vi "Dashboard Main.vi"() -> ()   [LabVIEW 2018]
uses:
  <vilib>/Utility/miscctls.llb/LVRowAndColumnTypeDef.ctl
  <vilib>/event_ctls.llb/eventvkey.ctl
  <vilib>/Rock Robotics/WPI/Dashboard/WPI_DashboardLogging Global.vi
  <vilib>/Rock Robotics/Network Tables/NT Read Boolean Array.vi
  <vilib>/Rock Robotics/Network Tables/NT Read Boolean.vi
panel:
  in  "TCP":refnum<k5>
  out "Robot IP":string
  out "Image Message":string="Timeout in Camera Communications"
  in  "Dashboard Tab":T1(tab)
  out "Boolean 17":bool
  out "Boolean 16":bool
  out "Boolean 15":bool
  out "Boolean 14":bool
  out "Boolean 13":bool
  out "Boolean 12":bool
  out "Boolean 11":bool
  out "Boolean 10":bool
  out "Boolean 9":bool
  out "Boolean 8":bool
  out "Boolean":bool
  out "Boolean":bool
  out "Boolean 6":bool
  out "Boolean 5":bool
  out "Boolean 4":bool
  out "Boolean 3":bool
  out "Boolean 2":bool
  out "Boolean":bool
  out "Elevator\nPosition":cluster{dbl, dbl}(slide) scale=0.0..22000.0
  out "Hatch Open":bool
  out "Hatch Close":bool
  out "Ball Out":bool
  out "Ball In":bool
  in  "Select Auto":string(combo)="Select Autonomous ..."
  out "NT Connection":bool
  out "Mode":T2(ring)=enum."Auto Disabled"
  out "Right Camera Perf":cluster{"Bandwidth (Mbps)":dbl, "FPS":dbl}
  in  "Rec Mode":enum32{"Stop", "Record", "Playback"}(radio)
  in  "Camera Name Right":string(combo)="No Camera Selection"
  in  "Camera Settings Right":T3={"Frame Rate"=30, "Compression"=30, "Size"=1, "DB Camera Config"=FALSE} {"Frame Rate" scale=1.0..30.0; "Compression" scale=100.0..-1.0; "Size" items=["640x480", "320x240", "160x120"]}
  in  "Camera Name":string(combo)="No Camera Selection"
  in  "Camera Settings":T3={"Frame Rate"=30, "Compression"=30, "Size"=1, "DB Camera Config"=FALSE} {"Frame Rate" scale=1.0..30.0; "Compression" scale=100.0..-1.0; "Size" items=["640x480", "320x240", "160x120"]}
  out "Camera Perf":string
  out "Boolean":bool
  out "Camera Image Right":T4(plugin-control)
  in  "DB/String 9":string
  in  "DB/String 8":string
  in  "DB/String 7":string
  in  "DB/String 6":string
  in  "DB/String 5":string
  in  "DB/String 4":string
  in  "DB/String 3":string
  in  "DB/String 2":string
  in  "DB/String 1":string
  in  "DB/String 0":string
  in  "DB/Slider 0":dbl(slide) scale=0.0..5.0
  in  "DB/Slider 1":dbl(slide) scale=0.0..5.0
  in  "DB/Slider 2":dbl(slide) scale=0.0..5.0
  in  "DB/Slider 3":dbl(slide) scale=0.0..5.0
  out "DB/LED 3":bool
  out "DB/LED 2":bool
  out "DB/LED 1":bool
  out "DB/LED 0":bool
  in  "DB/Button 3":bool
  in  "DB/Button 2":bool
  in  "DB/Button 1":bool
  in  "DB/Button 0":bool caption="New Name"
  in  "Test Slider":dbl(slide) scale=0.0..100.0 scale format="%#_3g"
  in  "On/Off":bool caption="Solenoid"
  in  "Test Name":u16(ring) items=["Select the test to run..."]
  in  "Test Tree":string(tree)
  in  "Motor":cluster{"Value":dbl, "Enable":bool} {"Value" scale=-1.0..1.0 scale format="%#_3g"}
  out "Progress":T5 {"Test Progress" scale=0.0..100.0}
  in  "Rev/Fwd":cluster{"Forward":bool, "Reverse":bool}
  in  "Test Ring":u16(ring) items=["Monochrome", "Color"]
  out "Cmd Status":string
  in  "Execute Command":bool
  in  "Command Params":string[][](table)
  in  "Command Selection":i32(listbox)
  in  "CheckList":i32(listbox)
  out "Tree":string(tree)
  out "Camera Image":T4(plugin-control)
  out "Background":bool
  # "Use this one"
  # "HW"
  # "HW"
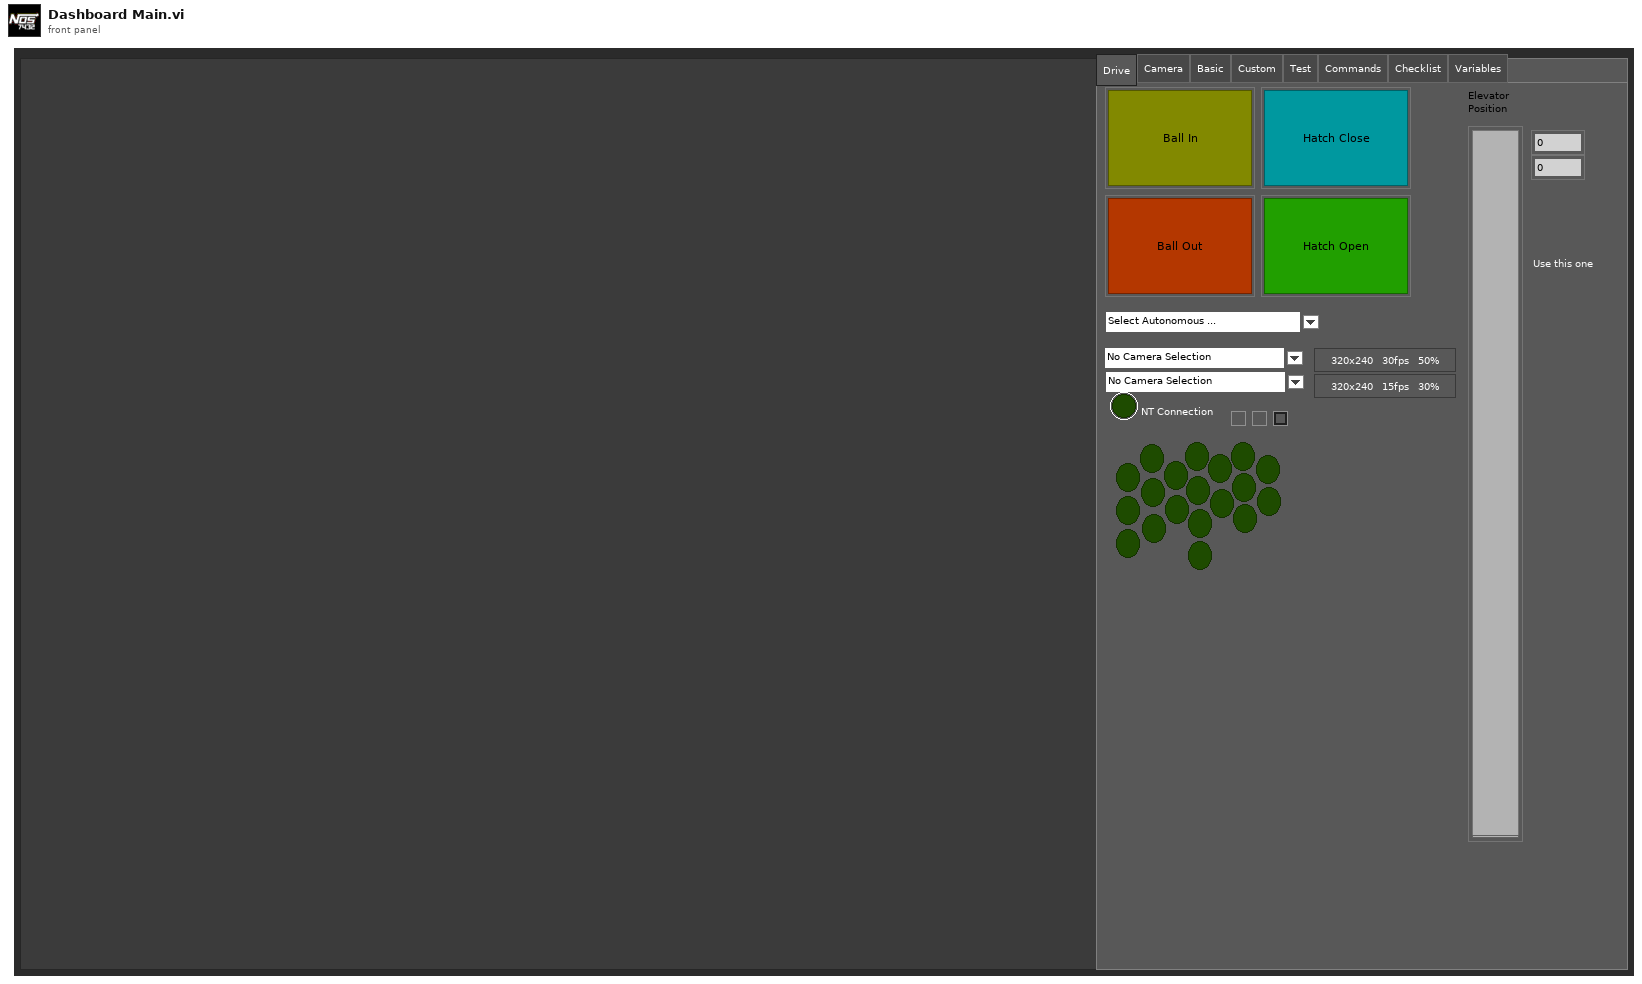
[diagram p1: front panel]
types:
  T1 = enum32{"Drive", "Camera", "Basic", "Custom", "Test", "Commands", "Checklist", "Variables"}
  T2 = enum8{"Tele-Op Disabled", "Tele-Op Enabled", "Auto Disabled", "Auto Enabled", "Test Disabled", "Test Enabled", "Disconnected", "No Code", "E-Stop"}
  T3 = cluster{"Frame Rate":i32, "Compression":i32, "Size":u16, "DB Camera Config":bool}
  T4 = typedef "IMAQ Image.ctl" = refnum<image>
  T5 = cluster{"Test Progress":u8, "Test Progress Text":string}
  T6 = cluster{"Save Path":path, "Interval (s)":dbl, "Keep":i32}
  T7 = typedef "Image Type" = u32
  T8 = cluster{"IDs":cluster{"RPC field ID":u16, "Unique ID":u16}, "String":string}
  T9 = cluster{"Error Strings":string, "Disable Counts":cluster{u16, u16}, "Rail Faults":cluster{u16, u16, u16}, "Robot IP":string, "DB Mode":u8, "Event Info":cluster{"Name":string, "Type":u8, "Number":u16, "Replay":u8}}
  T10 = cluster{"Storage":cluster{"Disk Free":u64, "RAM Block":u32, "RAM free":u32}, "CPU Utilization":cluster{"CPU % ISR":sgl, "CPU % Time Crit":sgl, "CPU % Timed Str":sgl, "CPU % High":sgl, "CPU % Above":sgl, "CPU % Normal":sgl, "CPU % Low":sgl}, "CAN":cluster{"% Bus Utilization":sgl, "Bus Off Cnt":u32, "TX_FIFO Full Cnt":u32, "Receive Error Cnt":u8, "Transmit Error Cnt":u8}, "HID":cluster{"HID Outputs":u32, "Rumble Low":u16, "Rumble High":u16}[]}
  T11 = cluster{"Status bits":cluster{"Test Mode":bool, "Autonomous":bool, "Enabled":bool, "Code Start":bool, "Brownout":bool, "Reserved 2":bool, "Reserved 3":bool, "E-Stop":bool}, "Code Trace":cluster{"Disabled":bool, "TeleOp":bool, "Auto":bool, "Test":bool}, "Controller Type":enum16{"unknown", "cRIO", "roboRio"}, "Code?":enum16{"unknown", "noCode", "code"}, "Battery V":dbl}
  T12 = cluster{"Control Bits":cluster{"TestMode":bool, "Autonomous":bool, "Enabled":bool, "FMS Present":bool, bool, bool, bool, "E-Stop":bool}, "Team Station ":u8, "Countdown":sgl, "Joystick Values":cluster{"Axes":dbl[], "Buttons":bool[], "POVs":i16[]}[]}
  T13 = cluster{"Global Rectangle":i32[], "Contours":cluster{"Contour Type":u32, "ROI Type":u32, "Points":i32[]}[]}
  T14 = cluster{"Camera Name":string, string, "Saved DB Images Info":cluster{"Save Path":path, "Interval (s)":dbl, "Keep":i32}}
  T15 = cluster{"Camera Name Right":string, string, "Saved DB Images Info":cluster{"Save Path":path, "Interval (s)":dbl, "Keep":i32}}
  T16 = cluster{"Operation":enum16{"Update", "Clear"}, "Color Box":u32}[]
  T17 = typedef "eventvkey.ctl" = enum16{"ASCII", "Enter", "Return", "Shift", "Ctrl", "Alt", "Cmd", "Opt", "Caps", "NumLock", "Clear", "Break", "Up", "Down", "Left", "Right", "Insert", "Delete", "Home", "End", "PageUp", "PageDown", "Escape", "Help", "Pause", "ScrollLock", "F1", "F2", "F3", "F4", "F5", "F6", "F7", "F8", "F9", "F10", "F11", "F12", "F13", "F14", "F15", "F16", "F17", "F18", "F19", "F20", "F21", "F22", "F23", "F24", "Play", "VolumeUp", "VolumeDown", "Mute", "Two Byte Char"}
  T18 = cluster{"Image Size":bool, "Image Type":bool, "Pixel Value":bool, "ROI Information":bool, "Zoom Factor":bool}
  T19 = cluster{"Operation":enum16{"Update", "Clear"}, "Color Box":u32}
  T20 = typedef "LVRowAndColumnTypeDef.ctl" = cluster{"Row":i32, "Column":i32}
  T21 = cluster{"Shift":bool, "Ctrl":bool, "Alt":bool, "Cmd":bool, "Opt":bool}
  T22 = typedef "imagedata.ctl" = cluster{"image type":i32, "image depth":i32, "image":u8[], "mask":u8[], "colors":u32[], "Rectangle":cluster{"left":i16, "top":i16, "right":i16, "bottom":i16}}
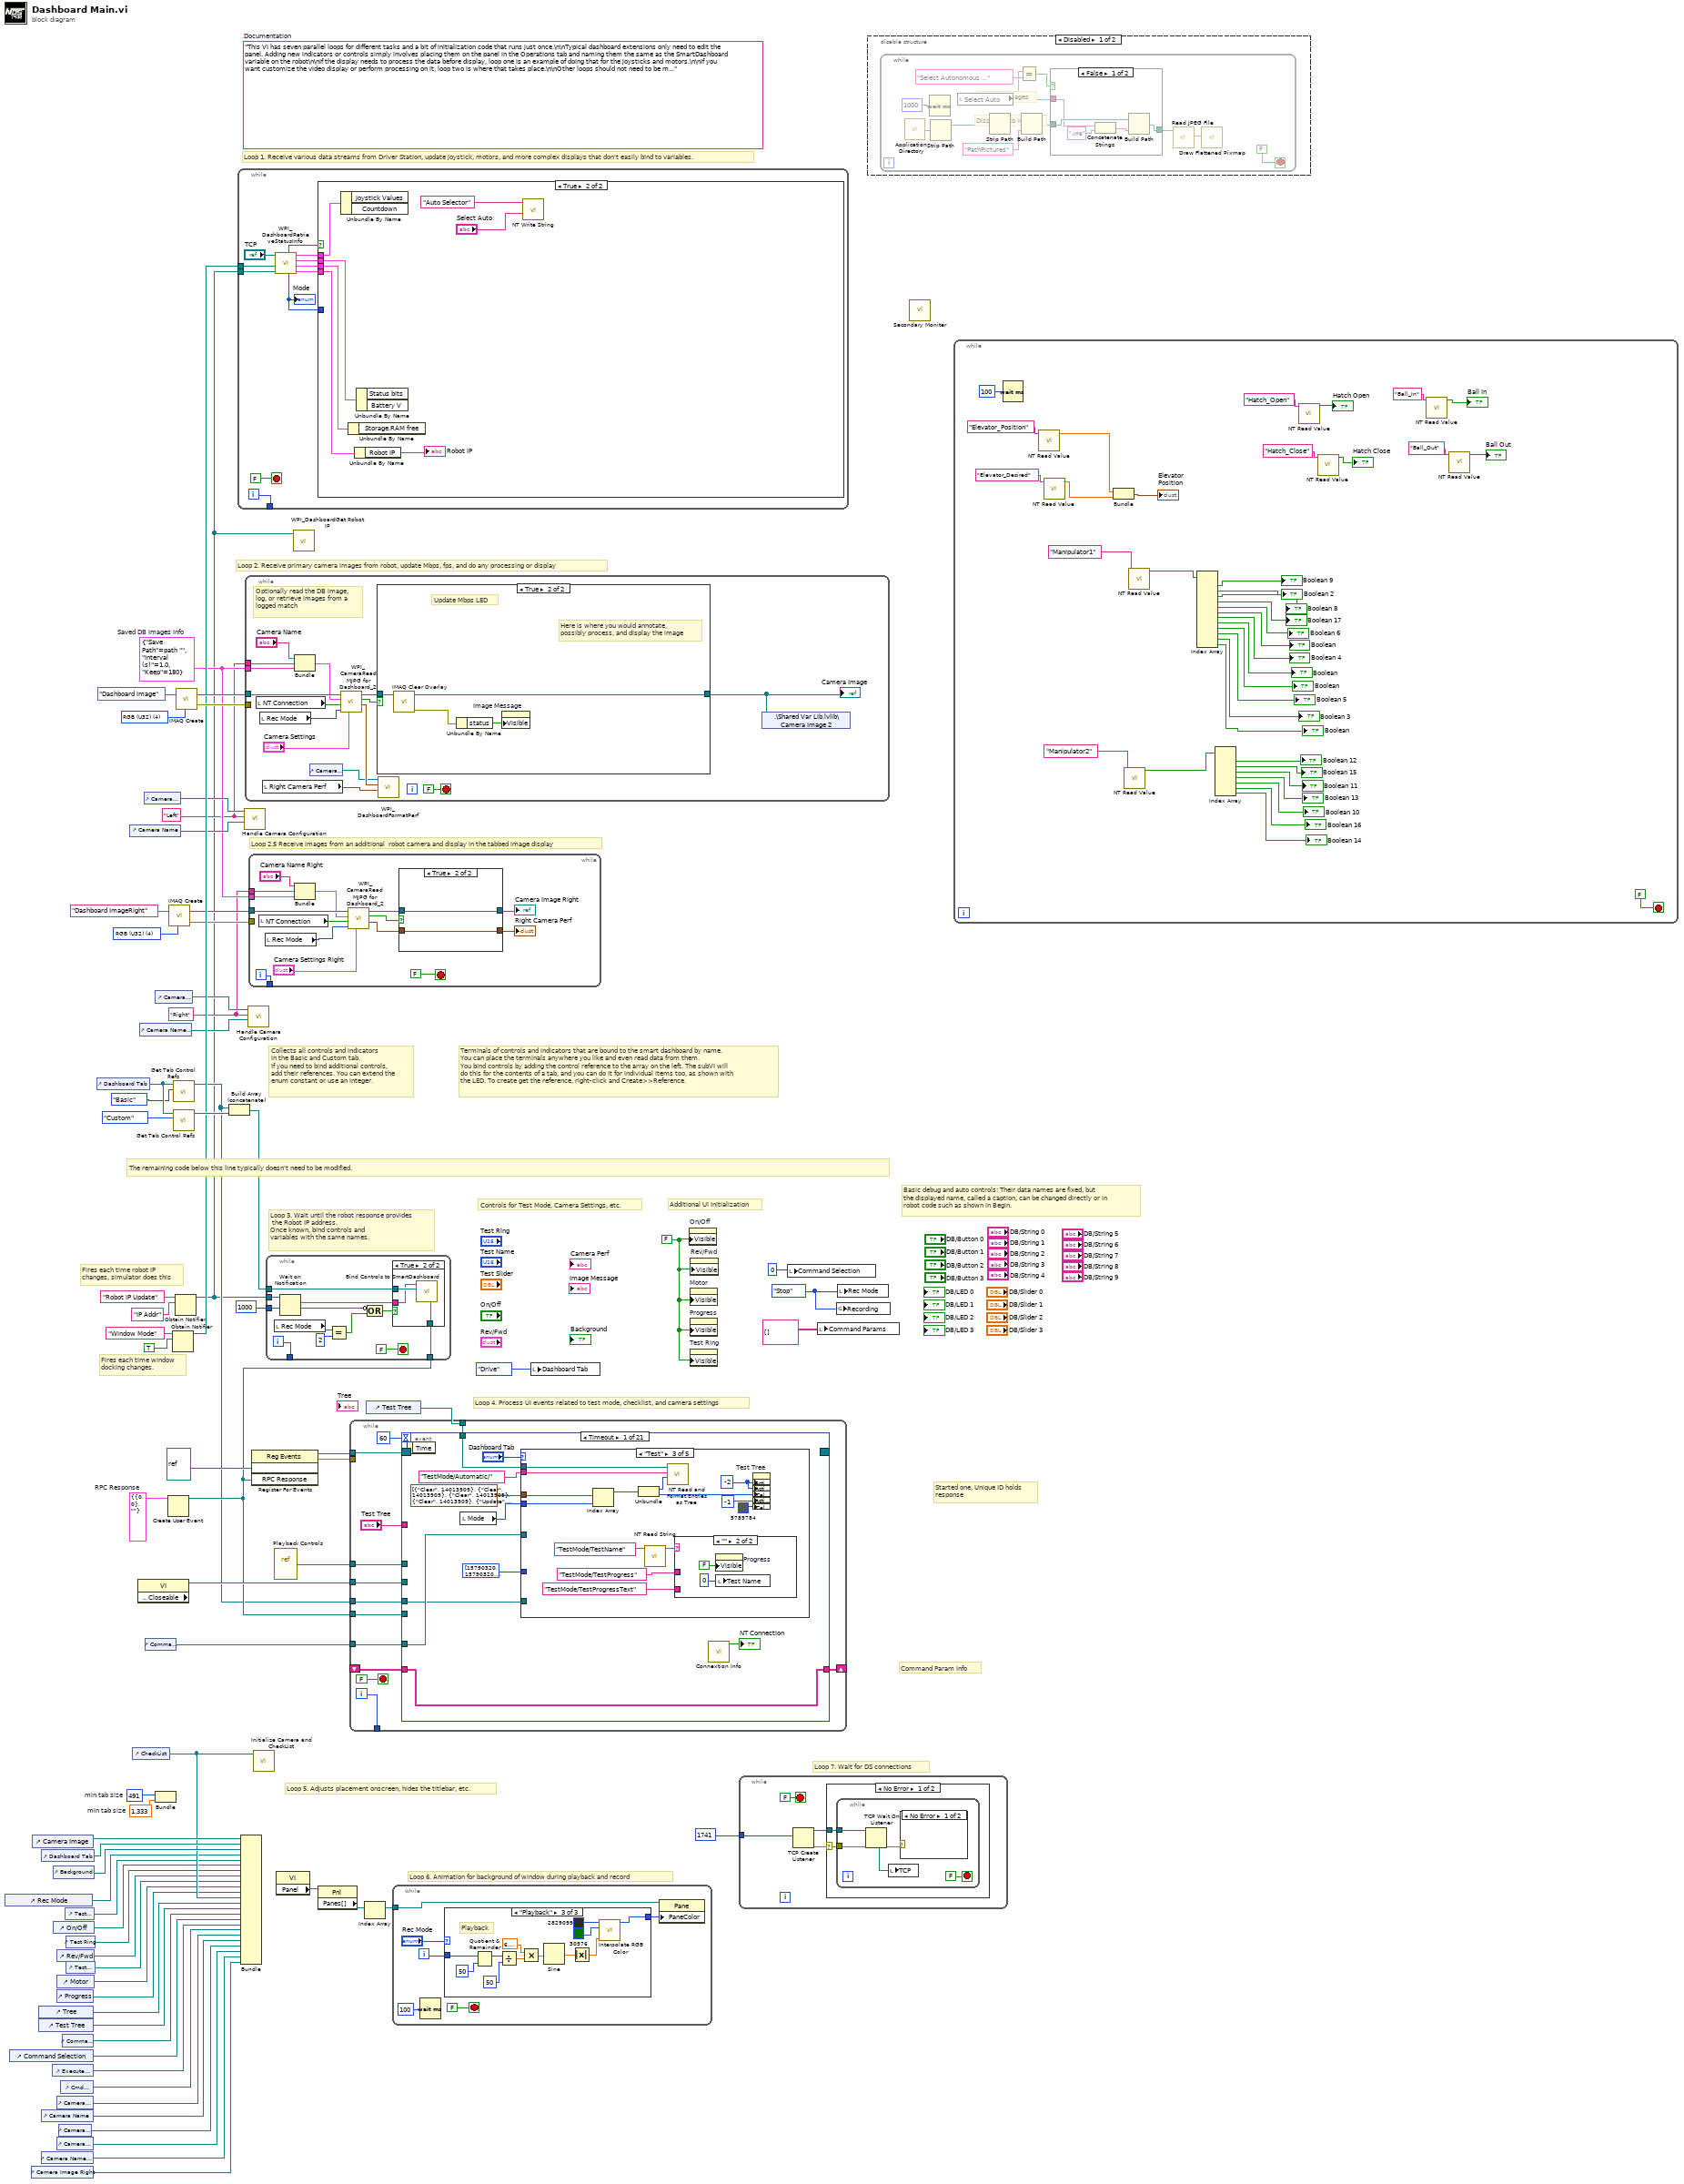
[diagram p0: block diagram]
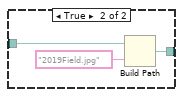
[diagram p2: hidden frame]
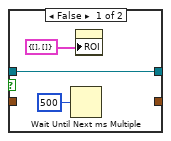
[diagram p4: hidden frame]
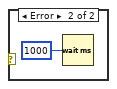
[diagram p5: hidden frame]
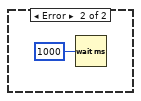
[diagram p6: hidden frame]
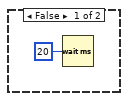
[diagram p7: hidden frame]
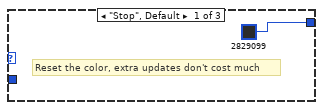
[diagram p8: hidden frame]
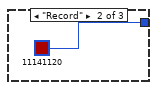
[diagram p9: hidden frame]
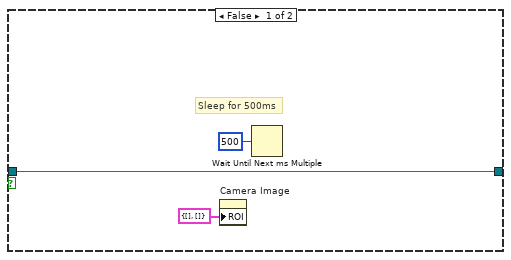
[diagram p11: hidden frame]
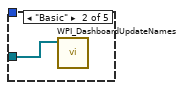
[diagram p13: hidden frame]
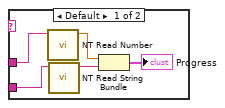
[diagram p14: hidden frame]
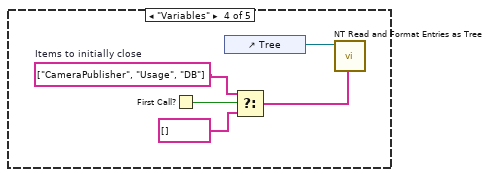
[diagram p15: hidden frame]
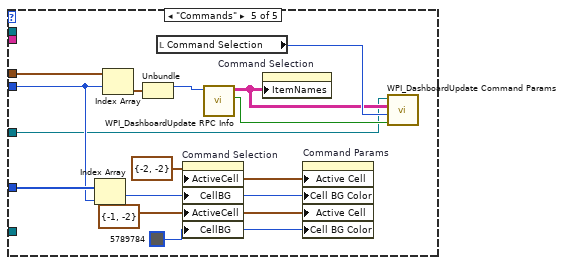
[diagram p16: hidden frame]
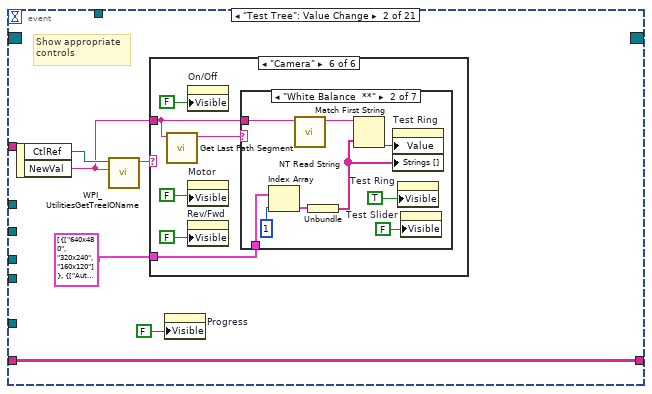
[diagram p17: hidden frame]
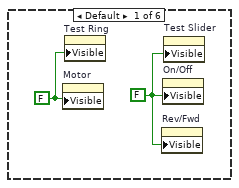
[diagram p18: hidden frame]
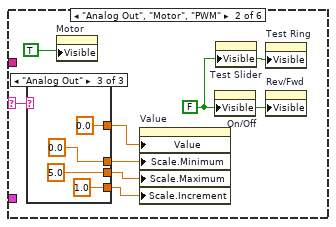
[diagram p19: hidden frame]
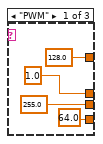
[diagram p20: hidden frame]
diagram:
  w4 = T6 {"Save Path"=path "", "Interval (s)"=1.0, "Keep"=180}  # Saved DB Images Info
  w3 = "Right"
  w2 = "Left"
  w14 = T7 4 items=["Grayscale (U8)", "Grayscale (I16)", "Grayscale (SGL)", "Complex (CSG)", "RGB (U32)", "HSL (U32)", "RGB (U64)"] ("Image Type")
  w28 = T8 {"IDs"={"RPC field ID"=0, "Unique ID"=0}, "String"=""}  # RPC Response
  w48 = 491  # min tab size
  w47 = 1.333  # min tab size
  w55 = enum32{"Stop", "Record", "Playback"}."Stop" ("Rec Mode")
  w34 = FALSE ("Visible")
  (unwired) "This VI has seven parallel loops for different tasks and a bit of initialization code that runs just once.\n\nTypical dashboard extensions only need to edit the panel. Adding new indicators or controls simply involves placing them on the panel in the Operations tab and naming them the same as the SmartDashboard variable on the robot\n\nIf the display needs to process the data before display, loop one is an example of doing that for the joysticks and motors.\n\nIf you want customize the video display or perform processing on it, loop two is where that takes place.\n\nOther loops should not need to be modified. They are pretty standard, and document the task they perform."  # Documentation
  w72 = T7 4 items=["Grayscale (U8)", "Grayscale (I16)", "Grayscale (SGL)", "Complex (CSG)", "RGB (U32)", "HSL (U32)", "RGB (U64)"] ("Image Type")
  # "300x300 images"
  # "Display Auto Image"
  # "Loop 2.5 Receive images from an additional  robot camera and display in the tabbed image display"
  # "Command Param Info"
  # "Started one, Unique ID holds\nresponse"
  # "Loop 7. Wait for DS connections"
  # "Basic debug and auto controls: Their data names are fixed, but\nthe displayed name, called a caption, can be changed directly or in\nrobot code such as shown in Begin."
  # "Controls for Test Mode, Camera Settings, etc."
  # "Additional UI Initialization"
  # "Loop 6. Animation for background of window during playback and record"
  # "Fires each time robot IP\nchanges, simulator does this"
  # "Fires each time window\ndocking changes."
  # "Collects all controls and indicators\nin the Basic and Custom tab.\nIf you need to bind additional controls,\nadd their references. You can extend the\nenum constant or use an integer."
  # "The remaining code below this line typically doesn't need to be modified."
  # "Loop 4. Process UI events related to test mode, checklist, and camera settings"
  # "Terminals of controls and indicators that are bound to the smart dashboard by name.\nYou can place the terminals anywhere you like and even read data from them.\nYou bind controls by adding the control reference to the array on the left. The subVI will\ndo this for the contents of a tab, and you can do it for individual items too, as shown with\nthe LED. To create get the reference, right-click and Create>>Reference."
  # "Loop 3. Wait until the robot response provides\n the Robot IP address.\nOnce known, bind controls and\nvariables with the same names."
  # "Loop 5. Adjusts placement onscreen, hides the titlebar, etc."
  # "Loop 1. Receive various data streams from Driver Station, update joystick, motors, and more complex displays that don't easily bind to variables."
  # "Loop 2. Receive primary camera images from robot, update Mbps, fps, and do any processing or display"
  n1 = control-ref of="Rec Mode"() -> (w40:refnum<vi>)
  n2 = control-ref of="Command Selection"() -> (w27:refnum<vi>)
  n3 = control-ref of="Camera Image Right"() -> (w7:refnum<vi>)
  n4 = control-ref of="Camera Image"() -> (w50:refnum<vi>)
  n5 = control-ref of="Tree"() -> (w44:refnum<vi>)
  n6 = control-ref of="Test Tree"() -> (w43:refnum<vi>)
  n7 = control-ref of="Dashboard Tab"() -> (w49:refnum<vi>)
  n8 = control-ref of="Camera Name"() -> (w18:refnum<vi>)
  n9 = control-ref of="Camera Name Right"() -> (w8:refnum<vi>)
  n10 = control-ref of="Execute Command"() -> (w29:refnum<vi>)
  n11 = control-ref of="Background"() -> (w46:refnum<vi>)
  n12 = control-ref of="On/Off"() -> (w38:refnum<vi>)
  n13 = control-ref of="Progress"() -> (w35:refnum<vi>)
  n14 = control-ref of="Camera Settings"() -> (w19:refnum<vi>)
  n15 = control-ref of="Camera Settings Right"() -> (w9:refnum<vi>)
  n16 = control-ref of="Rev/Fwd"() -> (w36:refnum<vi>)
  n17 = control-ref of="Motor"() -> (w41:refnum<vi>)
  n18 = control-ref of="Camera Perf"() -> (w17:refnum<vi>)
  n19 = control-ref of="Cmd Status"() -> (w23:refnum<vi>)
  n20 = control-ref of="Command Params"() -> (w30:refnum<vi>)
  n21 = control-ref of="Test Slider"() -> (w39:refnum<vi>)
  n22 = control-ref of="Test Ring"() -> (w37:refnum<vi>)
  n23 = control-ref of="Test Name"() -> (w42:refnum<vi>)
  n24 = control-ref of="Dashboard Tab"() -> (w53:refnum<vi>)
  n25 = control-ref of="Camera Name"() -> (w20:refnum<vi>)
  n26 = control-ref of="CheckList"() -> (w45:refnum<vi>)
  n27 = property class="VI" props=["Front Panel.Closeable"]() -> (reference out=w54:refnum<vi>)  [unwired: 2 in, 2 out]
  n28 = control-ref of="Camera Name Right"() -> (w10:refnum<vi>)
  n29 = control-ref of="Camera Settings"() -> (w21:refnum<vi>)
  n30 = control-ref of="Command Params"() -> (w22:refnum<vi>)
  n31 = control-ref of="Camera Settings Right"() -> (w11:refnum<vi>)
  n32 = Bundle("min tab size"=w48, "min tab size"=w47) -> ()  [unwired: 1 in, 1 out]
  n33 = Create User Event(user event datatype=w28) -> (user event=w24:refnum<user-event>)  [unwired: 1 in, 1 out]
  n34 = call "IMAQ Create"("Image Name"="Dashboard ImageRight", "Image Type"=w14) -> ("New Image"=w13:T4, "error out"=w12:errorcluster)  [unwired: 2 in, 1 out]
  n35 = Obtain Notifier(name (unnamed)="Window Mode", notification data type=TRUE) -> (notifier out=w33:refnum<notifier>)  [unwired: 2 in, 2 out]
  n36 = call <vilib>:"Get Tab Control Refs.vi"("Page Index"=T1."Basic" ("Dashboard Tab"), "TabControl in"=w53) -> ("ControlsOnPage"=w16:refnum<vi>[])  [unwired: 9 in]
  n37 = call <vilib>:"Get Tab Control Refs.vi"("Page Index"=T1."Custom" ("Dashboard Tab"), "TabControl in"=w53) -> ("ControlsOnPage"=w52:refnum<vi>[])  [unwired: 9 in]
  n38 = Obtain Notifier(name (unnamed)="Robot IP Update", notification data type="IP Addr" ("name (unnamed)")) -> (notifier out=w1:refnum<notifier>)  [unwired: 2 in, 2 out]
  n39 = call "IMAQ Create"("Image Name"="Dashboard Image", "Image Type"=w72) -> ("New Image"=w70:T4, "error out"=w69:errorcluster)  [unwired: 2 in, 1 out]
  n40 = Build Array (concatenate)(w16, w52) -> (w51:refnum<vi>[])
  n41 = while {
    tunnel: [w82] -> _
    tunnel: w1 -> [w76]
    tunnel: w33 -> [w73]
    i -> [w82]
    stop <- FALSE stop-if-true
    n42 = call <vilib>:"WPI_DashboardRetrieveStatusInfo.vi"("Binding Refnum"=w76, "Window Mode Notifier"=w73, "TCP Cnx"="TCP") -> ("Power and Errors"=w77:T9, "Robot Metrics"=w80:T10, "Status Info"=w81:T11, "Control Info"=w78:T12, "Robot Mode"=w75:T2, "Process?"=w79:bool)  [unwired: 3 in]
    "Mode" <- w75
    n43 = case shown="True" w79 {
      tunnel: w81 -> [_ w91]
      tunnel: w80 -> [_ w90]
      tunnel: w78 -> [_ w89]
      tunnel: w77 -> [_ w88]
      tunnel: w75 -> [_ _]
      frame False {
        n44 = Wait (ms)(milliseconds to wait=u32 20) -> ()  [unwired: 1 out]
      }
      frame True {
        n45 = Unbundle By Name(w89) -> ()  [unwired: 2 out]
        n46 = Unbundle By Name(w90) -> ()  [unwired: 1 out]
        n47 = Unbundle By Name(w88) -> ("Robot IP"=→"Robot IP":string)
        n48 = Unbundle By Name(w91) -> ()  [unwired: 2 out]
        n49 = call <vilib>:"NT Write String.vi"("String"="Select Auto", "Name"="Auto Selector") -> ()  [unwired: 9 in, 1 out]
      }
    }
  }
  n50 = Bundle("Camera Image"=w50, "Dashboard Tab"=w49, "Background"=w46, "Rec Mode"=w40, "Test Slider"=w39, "On/Off"=w38, "Test Ring"=w37, "Rev/Fwd"=w36, "Test Name"=w42, "Motor"=w41, "Progress"=w35, "CheckList"=w45, "Tree"=w44, "Test Tree"=w43, "Command Params"=w30, "Command Selection"=w27, "Execute Command"=w29, "Cmd Status"=w23, "Camera Settings"=w19, "Camera Name"=w18, "Camera Perf"=w17, "Camera Settings Right"=w9, "Camera Name Right"=w8, "Camera Image Right"=w7) -> ()  [unwired: 1 in, 1 out]
  n51 = call "Handle Camera Configuration.vi"("CameraNameRef"=w20, "Display Name"=w2, "ClusterRef"=w21) -> ()  [unwired: 9 in]
  n52 = while {
    tunnel: w70 -> [w105]
    tunnel: w69 -> [_]
    tunnel: w4 -> [w99]
    tunnel: w2 -> [w96]
    stop <- FALSE stop-if-true
    # "Optionally read the DB image,\nlog, or retrieve images from a\nlogged match"
    n53 = local read "NT Connection"() -> (w100:bool)
    n54 = local read "Rec Mode"() -> (w102:enum32{"Stop", "Record", "Playback"})
    n55 = local read "Right Camera Perf"() -> (w94:cluster{"Bandwidth (Mbps)":dbl, "FPS":dbl})
    n56 = Bundle("Camera Name"="Camera Name", w96, "Saved DB Images Info"=w99) -> (w98:T14)  [unwired: 1 in]
    n57 = control-ref of="Camera Perf"() -> (w93:refnum<vi>)
    n58 = call <vilib>:"WPI_CameraRead MJPG for Dashboard_2.vi"("Camera Settings"="Camera Settings", "Rec Mode"=w102, "NT Connection"=w100, "Capture Info"=w98, "Image in"=w105) -> ("perf info"=w95:cluster{"Bandwidth (Mbps)":dbl, "fps":dbl}, "Active"=w103:bool, "Image\\ out"=w104:T4)  [unwired: 4 in]
    n59 = case shown="True" w103 {
      tunnel: w104 -> [w108 w111]
      tunnel: [w108 w110] -> w92
      frame False {
        # "Sleep for 500ms"
        n60 = property on="Camera Image" class="ImageControl"("ROI"=T13 {"Global Rectangle"=[], "Contours"=[]}) -> ()  [unwired: 2 in, 2 out]
        n61 = Wait Until Next ms Multiple(millisecond multiple=u32 500) -> ()  [unwired: 1 out]
      }
      frame True {
        # "Here is where you would annotate,\npossibly process, and display the image"
        # "Update Mbps LED"
        n62 = call "IMAQ Clear Overlay"("Image"=w111) -> ("error out"=w112:errorcluster, "Image Out"=w110:T4)  [unwired: 2 in, 7 out]
        n63 = Unbundle By Name(w112) -> ("status"=w113:bool)
        n64 = property on="Image Message" class="Str"("Visible"=w113) -> ()  [unwired: 2 in, 2 out]
      }
    }
    "Camera Image" <- w92
    n65 = call <vilib>:"WPI_DashboardFormatPerf.vi"("Right Camera Perf"=w94, "Performance"=w95, "String in"=w93) -> ()  [unwired: 9 in]
    n66 = shared-variable ".\\Shared Var Lib.lvlib\\Camera Image 2"(w92) -> ()  [unwired: 1 in, 1 out]
  }
  n67 = call "Handle Camera Configuration.vi"("CameraNameRef"=w10, "Display Name"=w3, "ClusterRef"=w11) -> ()  [unwired: 9 in]
  n68 = while {
    tunnel: w13 -> [w128]
    tunnel: w12 -> [_]
    tunnel: [w123] -> _
    tunnel: w4 -> [w119]
    tunnel: w3 -> [w116]
    i -> [w123]
    stop <- FALSE stop-if-true
    n69 = local read "NT Connection"() -> (w120:bool)
    n70 = local read "Rec Mode"() -> (w127:enum32{"Stop", "Record", "Playback"})
    n71 = Bundle("Camera Name Right"="Camera Name Right", w116, "Saved DB Images Info"=w119) -> (w118:T15)  [unwired: 1 in]
    n72 = call <vilib>:"WPI_CameraRead MJPG for Dashboard_2.vi"("Camera Settings"="Camera Settings Right", "Rec Mode"=w127, "NT Connection"=w120, "Capture Info"=w118, "Image in"=w128) -> ("perf info"=w114:cluster{"Bandwidth (Mbps)":dbl, "fps":dbl}, "Active"=w122:bool, "Image\\ out"=w125:T4)  [unwired: 4 in]
    n73 = case shown="True" w122 {
      tunnel: w125 -> [w130 w133]
      tunnel: [w130 w133] -> w121
      tunnel: [_ w132] -> w115
      tunnel: w114 -> [_ w132]
      frame False {
        n74 = Wait Until Next ms Multiple(millisecond multiple=u32 500) -> ()  [unwired: 1 out]
        n75 = property on="Camera Image Right" class="ImageControl"("ROI"=T13 {"Global Rectangle"=[], "Contours"=[]}) -> ()  [unwired: 2 in, 2 out]
      }
      frame True {
      }
    }
    "Camera Image Right" <- w121
    "Right Camera Perf" <- w115
  }
  n76 = register-events(refnum<vi> refnum, w24) -> (reference out=w59:refnum<event-registration>, error out=w58:errorcluster)  [unwired: 2 in]
  n77 = call "Initialize Camera and CheckList.vi"("ListBox in"=w45) -> ()  [unwired: 11 in]
  n78 = while {
    tunnel: w51 -> [w145]
    tunnel: w1 -> [w143]
    tunnel: [w141] -> _
    tunnel: u32 1000 ("milliseconds to wait") -> [w140]
    tunnel: w24 -> [w134]
    i -> [w141]
    stop <- FALSE stop-if-true
    n79 = local read "Rec Mode"() -> (w136:enum32{"Stop", "Record", "Playback"})
    n80 = Wait on Notification(notifier=w143, timeout in ms (-1)=w140) -> (notification=w142:string, timed out?=w138:bool)  [unwired: 2 in, 2 out]
    n81 = Equal?(x=w136, y=u16 2 ("Rec Mode")) -> (x = y?=w137:bool)
    n82 = Compound Arithmetic op=OR(invert w138, w137) -> (w139:bool)
    n83 = case shown="True" w139 {
      tunnel: w145 -> [_ w148]
      tunnel: w142 -> [_ w147]
      tunnel: w134 -> [_ w146]
      frame False {
      }
      frame True {
        n84 = call <vilib>:"Bind Controls to SmartDashboard.vi"("RPC ref"=w146, "Bound Control Refs"=w148, "Server IP Address"=w147) -> ()  [unwired: 9 in]
      }
    }
  }
  n85 = vi-ref "Playback Controls.vi"() -> (w60:refnum<vi>)
  n86 = property class="VI"() -> ("Panel"=w62:refnum<vi>)  [unwired: 2 in, 2 out]
  n87 = call "WPI_DashboardGet Robot IP.vi"("Notifier in"=w1) -> ()  [unwired: 11 in]
  n88 = property class="Pnl"(reference=w62) -> ("Panes[]"=w63:refnum<vi>[])  [unwired: 1 in, 2 out]
  n89 = Index Array(array=w63) -> (element=w61:refnum<vi>)  [unwired: 1 in]
  n90 = control-ref of="Test Tree"() -> (w64:refnum<vi>)
  n91 = while {
    tunnel: [w158] -> _
    tunnel: w64 -> [w157]
    tunnel: w60 -> [w156]
    tunnel: w59 -> [w155]
    tunnel: w58 -> [_]
    tunnel: w54 -> [w154]
    tunnel: w24 -> [w153]
    tunnel: w22 -> [w152]
    shift-right: [w151] -> _
    shift-left: _ -> [w150]
    tunnel: w16 -> [w149]
    i -> [w158]
    stop <- FALSE stop-if-true
    n92 = event shown="[0] Timeout" {
      selector: w155 -> [_ _ _ _ _ _ _ _ _ _ _ _ _ _ _ _ _ _ _ _ _]
      dyn-events: [_ _ _ _ _ _ _ _ _ _ _ _ _ _ _ _ w418 _ _ _ _] -> _
      timeout: u32 60 ("milliseconds to wait") -> [_ _ _ _ _ _ _ _ _ _ _ _ _ _ _ _ _ _ _ _ _]
      tunnel: w157 -> [w170 _ _ _ _ _ _ _ _ _ _ _ _ _ _ _ _ _ _ _ _]
      tunnel: "Test Tree" -> [_ _ _ _ _ _ _ _ _ _ _ w385 w393 w395 w399 w407 _ _ _ _ _]
      tunnel: w156 -> [_ _ _ _ _ _ _ _ _ _ _ _ _ _ _ _ w420 _ w438 _ _]
      tunnel: w154 -> [_ _ _ _ _ _ _ _ _ _ _ _ _ _ _ _ w416 _ _ _ _]
      tunnel: w153 -> [_ _ _ _ _ _ _ _ _ _ _ _ _ _ _ _ w414 _ _ _ _]
      tunnel: w152 -> [w165 _ _ _ _ _ w336 _ _ _ _ _ _ _ _ _ _ _ _ _ _]
      tunnel: [w164 w213 w315 w320 w329 w333 w334 w343 w353 w360 w372 w384 w391 w394 w398 w406 w413 w433 w435 w439 w452] -> w151
      tunnel: w150 -> [w164 w213 w315 w320 w329 w333 w334 _ _ w360 w372 w384 w391 w394 w398 w406 w413 w433 w435 w439 w452]
      tunnel: w149 -> [w162 _ _ _ _ _ _ _ _ _ _ _ _ _ _ _ _ _ _ _ _]
      event Timeout {
        n93 = event-data() -> ()  [unwired: 1 in, 1 out]
        n94 = local read "Mode"() -> (w167:T2)
        n95 = case shown="\"Test\"" "Dashboard Tab" {
          tunnel: w170 -> [_ _ w186 _ _]
          tunnel: "TestMode/Automatic/" ("Name Pattern") -> [_ _ w185 _ _]
          tunnel: T16 [{"Operation"=enum."Clear", "Color Box"=14013909}, {"Operation"=enum."Clear", "Color Box"=14013909}, {"Operation"=enum."Clear", "Color Box"=14013909}, {"Operation"=enum."Clear", "Color Box"=14013909}, {"Operation"=enum."Update", "Color Box"=14013909}, {"Operation"=enum."Update", "Color Box"=16777215}, {"Operation"=enum."Clear", "Color Box"=14013909}, {"Operation"=enum."Clear", "Color Box"=14013909}, {"Operation"=enum."Clear", "Color Box"=14013909}] -> [_ _ w178 _ w206]
          tunnel: w167 -> [_ _ w177 _ w205]
          tunnel: u32[] [15790320, 15790320, 15790320, 15790320, 16777215, 16777215, 15790320, 15790320, 15790320] -> [_ _ _ _ w211]
          tunnel: w165 -> [_ _ _ _ w199]
          tunnel: w162 -> [_ w172 _ _ _]
          frame "Custom", Default {
          }
          frame "Basic" {
            n96 = call <vilib>:"WPI_DashboardUpdateNames.vi"("Controls on Tab"=w172) -> ()  [unwired: 11 in]
          }
          frame "Test" {
            w184 = -2 ("Active Item:Row Number")
            n97 = Index Array(array=w178, index=w177) -> (element=w179:T19)
            n98 = Unbundle(w179) -> ("Operation"=w180:enum16{"Update", "Clear"}, "Color Box"=w181:u32)
            n99 = call <vilib>:"NT Read String.vi"("Name"="TestMode/TestName") -> ("String"=w175:string)  [unwired: 9 in, 1 out]
            n100 = call <vilib>:"NT Read and Format Entries as Tree.vi"("Operation"=w180, "Name Pattern"=w185, "Tree Refnum"=w186) -> ()  [unwired: 7 in, 2 out]
            n101 = case shown="\"\"" w175 {
              tunnel: "TestMode/TestProgress" ("Name") -> [w188 _]
              tunnel: "TestMode/TestProgressText" ("Name") -> [w187 _]
              frame Default {
                n102 = call <vilib>:"NT Read Number.vi"("Name"=w188) -> ("Numeric"=w189:dbl)  [unwired: 9 in, 1 out]
                n103 = call <vilib>:"NT Read String.vi"("Name"=w187) -> ("String"=w190:string)  [unwired: 9 in, 1 out]
                n104 = Bundle("Numeric"=w189, "String"=w190) -> (→"Progress":cluster{"Numeric":dbl, "String":string})  [unwired: 1 in]
              }
              frame "" {
                n105 = property on="Progress" class="Clust (strict)"("Visible"=FALSE) -> ()  [unwired: 2 in, 2 out]
                n106 = local write "Test Name"(u16 0) -> ()
              }
            }
            n107 = property on="Test Tree" class="Tree (strict)"("Active Item Row Number"=w184, "ActiveColNum"=w184, "CellBG"=w181, "Active Item Row Number"=-1 ("Active Item:Row Number"), "CellBG"=u32 5789784 ("Color Box")) -> ()  [unwired: 2 in, 2 out]
          }
          frame "Variables" {
            w196 = string[] ["CameraPublisher", "Usage", "DB"]  # Items to initially close
            n108 = First Call?() -> (First Call?: T/F=w197:bool)
            n109 = control-ref of="Tree"() -> (w198:refnum<vi>)
            n110 = Select(t=w196, s=w197, f=string[] []) -> (s? t:f=w194:string[])
            n111 = call <vilib>:"NT Read and Format Entries as Tree.vi"("Tags to  Close"=w194, "Tree Refnum"=w198) -> ()  [unwired: 8 in, 2 out]
          }
          frame "Commands" {
            w207 = u32 5789784 ("Color Box")
            w208 = T20 {"Row"=-1, "Column"=-2} ("Active Cell:Active Cell")
            w210 = T20 {"Row"=-2, "Column"=-2} ("Active Cell:Active Cell")
            n112 = Index Array(array=w211, index=w205) -> (element=w209:u32)
            n113 = Index Array(array=w206, index=w205) -> (element=w204:T19)
            n114 = Unbundle(w204) -> ("Operation"=w203:enum16{"Update", "Clear"})  [unwired: 1 out]
            n115 = local read "Command Selection"() -> (w202:i32)
            n116 = property on="Command Selection" class="MCListbox (strict)"("ActiveCell"=w210, "CellBG"=w209, "ActiveCell"=w208, "CellBG"=w207) -> ()  [unwired: 2 in, 2 out]
            n117 = call <vilib>:"WPI_DashboardUpdate RPC Info.vi"("Operation"=w203) -> ("update"=w201:bool, "commands"=w200:string[][])  [unwired: 9 in]
            n118 = property on="Command Selection" class="MCListbox (strict)"("ItemNames"=w200) -> ()  [unwired: 2 in, 2 out]
            n119 = property on="Command Params" class="Tbl (strict)"("Active Cell"=w210, "Cell BG Color"=w209, "Active Cell"=w208, "Cell BG Color"=w207) -> ()  [unwired: 2 in, 2 out]
            n120 = call <vilib>:"WPI_DashboardUpdate Command Params.vi"("Update"=w201, "NewVal"=w202, "Commands"=w200, "Param Tbl"=w199) -> ()  [unwired: 7 in, 1 out]
          }
        }
        n121 = call <vilib>:"Connextion Info.vi"() -> ("Connected"=→"NT Connection":bool)  [unwired: 10 in, 1 out]
      }
      event "Test Tree": Value Change {
        # "Show appropriate\ncontrols"
        n122 = event-data() -> ("CtlRef"=w216:refnum<vi>, "NewVal"=w214:string)  [unwired: 1 in]
        n123 = call <vilib>:"WPI_UtilitiesGetTreeIOName.vi"("NewVal"=w214, "TreeControl in"=w216) -> ("I/O Name"=w217:string)  [unwired: 9 in]
        n124 = case shown="\"Camera\"" w217 {
          selector: w217 -> [_ w224 _ w246 w255 _]
          tunnel: w214 -> [_ _ w243 w245 _ w262]
          tunnel: cluster{string[]}[] [{["640x480", "320x240", "160x120"]}, {["Auto", "Fixed indoor", "Fixed outdoor 1", "Fixed outdoor 2", "Fixed fluorescent 1", "Fixed fluorescent 2", "Hold current"]}, {["Auto", "Flicker-free 50 Hz", "Flicker-free 60 Hz", "Hold current"]}, {["None", "Prioritize frame rate", "Prioritize image quality"]}, {["Monochrome", "Color"]}] -> [_ _ _ _ _ w261]
          frame Default {
            w219 = FALSE ("Visible")
            w218 = FALSE ("Visible")
            n125 = property on="Motor" class="Clust (strict)"("Visible"=w218) -> ()  [unwired: 2 in, 2 out]
            n126 = property on="Test Ring" class="Ring (strict)"("Visible"=w218) -> ()  [unwired: 2 in, 2 out]
            n127 = property on="Rev/Fwd" class="Clust (strict)"("Visible"=w219) -> ()  [unwired: 2 in, 2 out]
            n128 = property on="On/Off" class="Bool (strict)"("Visible"=w219) -> ()  [unwired: 2 in, 2 out]
            n129 = property on="Test Slider" class="Slide (strict)"("Visible"=w219) -> ()  [unwired: 2 in, 2 out]
          }
          frame "Analog Out", "Motor", "PWM" {
            w225 = FALSE ("Visible")
            n130 = case shown="\"Analog Out\"" w224 {
              tunnel: [1.0 ("Value") -1.0 ("Value") 0.0 ("Value")] -> w223
              tunnel: [255.0 ("Value") 1.0 ("Value") 5.0 ("Value")] -> w222
              tunnel: [128.0 ("Value") 0.0 ("Value") 0.0 ("Value")] -> w221
              tunnel: [64.0 ("Value") 0.5 ("Value") 1.0 ("Value")] -> w220
              frame "PWM" {
              }
              frame "Motor", Default {
              }
              frame "Analog Out" {
              }
            }
            n131 = property on="Motor" class="Clust (strict)"("Visible"=TRUE) -> ()  [unwired: 2 in, 2 out]
            n132 = property on="Value" class="Slide (strict)"("Value"=w221, "Scale.Minimum"=w223, "Scale.Maximum"=w222, "Scale.Increment"=w220) -> ()  [unwired: 2 in, 2 out]
            n133 = property on="On/Off" class="Bool (strict)"("Visible"=w225) -> ()  [unwired: 2 in, 2 out]
            n134 = property on="Test Slider" class="Slide (strict)"("Visible"=w225) -> ()  [unwired: 2 in, 2 out]
            n135 = property on="Test Ring" class="Ring (strict)"("Visible"=w225) -> ()  [unwired: 2 in, 2 out]
            n136 = property on="Rev/Fwd" class="Clust (strict)"("Visible"=w225) -> ()  [unwired: 2 in, 2 out]
          }
          frame "Servo" {
            w241 = FALSE ("Visible")
            n137 = call <vilib>:"NT Read Number.vi"("Name"=w243) -> ("Numeric"=w242:dbl)  [unwired: 9 in, 1 out]
            n138 = property on="Test Slider" class="Slide (strict)"("Visible"=TRUE, "Scale.Maximum"=170.0 ("Scale.Range:Maximum")) -> ()  [unwired: 2 in, 2 out]
            n139 = local write "Test Slider"(w242) -> ()
            n140 = property on="Motor" class="Clust (strict)"("Visible"=w241) -> ()  [unwired: 2 in, 2 out]
            n141 = property on="Rev/Fwd" class="Clust (strict)"("Visible"=w241) -> ()  [unwired: 2 in, 2 out]
            n142 = property on="On/Off" class="Bool (strict)"("Visible"=w241) -> ()  [unwired: 2 in, 2 out]
            n143 = property on="Test Ring" class="Ring (strict)"("Visible"=w241) -> ()  [unwired: 2 in, 2 out]
          }
          frame "Relay", "Solenoid" {
            w244 = FALSE ("Visible")
            n144 = property on="Motor" class="Clust (strict)"("Visible"=w244) -> ()  [unwired: 2 in, 2 out]
            n145 = property on="Test Slider" class="Slide (strict)"("Visible"=w244) -> ()  [unwired: 2 in, 2 out]
            n146 = Search and Replace String(input string=w245, search string="/Value  **", replace string="/Direction") -> (result string=w251:string)  [unwired: 5 in, 3 out]
            n147 = property on="Test Ring" class="Ring (strict)"("Visible"=w244) -> ()  [unwired: 2 in, 2 out]
            n148 = call <vilib>:"NT Read String.vi"("Name"=w251) -> ("String"=w249:string)  [unwired: 9 in, 1 out]
            n149 = Equal?(x="Both directions", y=w249) -> (x = y?=w247:bool)
            n150 = Not(x=w247) -> (.not. x?=w248:bool)
            n151 = property on="Rev/Fwd" class="Clust (strict)"("Visible"=w247) -> ()  [unwired: 2 in, 2 out]
            n152 = property on="On/Off" class="Bool (strict)"("Visible"=w248, "Caption.Text"=w246) -> ()  [unwired: 2 in, 2 out]
          }
          frame "Compressor", "Digital Out" {
            w254 = FALSE ("Visible")
            # "Get direction and finish"
            n153 = property on="Motor" class="Clust (strict)"("Visible"=w254) -> ()  [unwired: 2 in, 2 out]
            n154 = property on="Test Slider" class="Slide (strict)"("Visible"=w254) -> ()  [unwired: 2 in, 2 out]
            n155 = property on="Test Ring" class="Ring (strict)"("Visible"=w254) -> ()  [unwired: 2 in, 2 out]
            n156 = property on="On/Off" class="Bool (strict)"("Visible"=TRUE, "Caption.Text"=w255) -> ()  [unwired: 2 in, 2 out]
            n157 = property on="Rev/Fwd" class="Clust (strict)"("Visible"=FALSE) -> ()  [unwired: 2 in, 2 out]
          }
          frame "Camera" {
            n158 = call <vilib>:"Get Last Path Segment.vi"("String in"=w262) -> ("String out"=w263:string)  [unwired: 10 in]
            n159 = property on="On/Off" class="Bool (strict)"("Visible"=FALSE) -> ()  [unwired: 2 in, 2 out]
            n160 = property on="Motor" class="Clust (strict)"("Visible"=FALSE) -> ()  [unwired: 2 in, 2 out]
            n161 = property on="Rev/Fwd" class="Clust (strict)"("Visible"=FALSE) -> ()  [unwired: 2 in, 2 out]
            n162 = case shown="\"White Balance  **\"" w263 {
              tunnel: w262 -> [w269 w278 w287 w296 w305 _ w311]
              tunnel: w261 -> [w267 w275 w284 w293 w302 _ _]
              frame "Size  **" {
                n163 = Index Array(array=w267) -> (element=w266:cluster{string[]})  [unwired: 1 in]
                n164 = call <vilib>:"NT Read String.vi"("Name"=w269) -> ("String"=w268:string)  [unwired: 9 in, 1 out]
                n165 = Unbundle(w266) -> (w264:string[])
                n166 = Match First String(2:w264, 3:w268) -> (0:w265:i32)  [unwired: 1 out]
                n167 = property on="Test Ring" class="Ring (strict)"("Value"=w265, "Strings []"=w264) -> ()  [unwired: 2 in, 2 out]
                n168 = property on="Test Ring" class="Ring (strict)"("Visible"=TRUE) -> ()  [unwired: 2 in, 2 out]
                n169 = property on="Test Slider" class="Slide (strict)"("Visible"=FALSE) -> ()  [unwired: 2 in, 2 out]
              }
              frame "White Balance  **" {
                n170 = Index Array(array=w275, index=1) -> (element=w276:cluster{string[]})
                n171 = call <vilib>:"NT Read String.vi"("Name"=w278) -> ("String"=w277:string)  [unwired: 9 in, 1 out]
                n172 = Unbundle(w276) -> (w273:string[])
                n173 = Match First String(2:w273, 3:w277) -> (0:w272:i32)  [unwired: 1 out]
                n174 = property on="Test Ring" class="Ring (strict)"("Value"=w272, "Strings []"=w273) -> ()  [unwired: 2 in, 2 out]
                n175 = property on="Test Ring" class="Ring (strict)"("Visible"=TRUE) -> ()  [unwired: 2 in, 2 out]
                n176 = property on="Test Slider" class="Slide (strict)"("Visible"=FALSE) -> ()  [unwired: 2 in, 2 out]
              }
              frame "Exposure  **" {
                n177 = Index Array(array=w284, index=2) -> (element=w285:cluster{string[]})
                n178 = call <vilib>:"NT Read String.vi"("Name"=w287) -> ("String"=w286:string)  [unwired: 9 in, 1 out]
                n179 = Unbundle(w285) -> (w281:string[])
                n180 = Match First String(2:w281, 3:w286) -> (0:w282:i32)  [unwired: 1 out]
                n181 = property on="Test Ring" class="Ring (strict)"("Value"=w282, "Strings []"=w281) -> ()  [unwired: 2 in, 2 out]
                n182 = property on="Test Ring" class="Ring (strict)"("Visible"=TRUE) -> ()  [unwired: 2 in, 2 out]
                n183 = property on="Test Slider" class="Slide (strict)"("Visible"=FALSE) -> ()  [unwired: 2 in, 2 out]
              }
              frame "Exposure Priority  **" {
                n184 = Index Array(array=w293, index=3) -> (element=w294:cluster{string[]})
                n185 = call <vilib>:"NT Read String.vi"("Name"=w296) -> ("String"=w295:string)  [unwired: 9 in, 1 out]
                n186 = Unbundle(w294) -> (w290:string[])
                n187 = Match First String(2:w290, 3:w295) -> (0:w291:i32)  [unwired: 1 out]
                n188 = property on="Test Ring" class="Ring (strict)"("Value"=w291, "Strings []"=w290) -> ()  [unwired: 2 in, 2 out]
                n189 = property on="Test Ring" class="Ring (strict)"("Visible"=TRUE) -> ()  [unwired: 2 in, 2 out]
                n190 = property on="Test Slider" class="Slide (strict)"("Visible"=FALSE) -> ()  [unwired: 2 in, 2 out]
              }
              frame "Color Enable  **" {
                n191 = Index Array(array=w302, index=4) -> (element=w303:cluster{string[]})
                n192 = call <vilib>:"NT Read String.vi"("Name"=w305) -> ("String"=w304:string)  [unwired: 9 in, 1 out]
                n193 = Unbundle(w303) -> (w299:string[])
                n194 = Match First String(2:w299, 3:w304) -> (0:w300:i32)  [unwired: 1 out]
                n195 = property on="Test Ring" class="Ring (strict)"("Value"=w300, "Strings []"=w299) -> ()  [unwired: 2 in, 2 out]
                n196 = property on="Test Ring" class="Ring (strict)"("Visible"=TRUE) -> ()  [unwired: 2 in, 2 out]
                n197 = property on="Test Slider" class="Slide (strict)"("Visible"=FALSE) -> ()  [unwired: 2 in, 2 out]
              }
              frame Default {
                n198 = property on="Test Ring" class="Ring (strict)"("Visible"=FALSE) -> ()  [unwired: 2 in, 2 out]
                n199 = property on="Test Slider" class="Slide (strict)"("Visible"=FALSE) -> ()  [unwired: 2 in, 2 out]
              }
              frame "Brightness  **", "Color Level  **", "Compression  **", "FPS  **", "Sharpness  **" {
                n200 = call <vilib>:"NT Read Number.vi"("Name"=w311) -> ("Numeric"=w310:dbl)  [unwired: 9 in, 1 out]
                n201 = local write "Test Slider"(w310) -> ()
                n202 = property on="Test Slider" class="Slide (strict)"("Visible"=TRUE, "Scale.Maximum"=100.0 ("Scale.Range:Maximum")) -> ()  [unwired: 2 in, 2 out]
                n203 = property on="Test Ring" class="Ring (strict)"("Visible"=FALSE) -> ()  [unwired: 2 in, 2 out]
              }
            }
          }
        }
        n204 = property on="Progress" class="Clust (strict)"("Visible"=FALSE) -> ()  [unwired: 2 in, 2 out]
      }
      event "Test Name": Mouse Enter {
        # "Populate the ring with the list of tests"
        n205 = event-data() -> ()  [unwired: 1 in, 1 out]
        n206 = call <vilib>:"NT Read String Array.vi"("Name"="TestMode/TestList") -> ("String Array"=w319:string[])  [unwired: 9 in, 1 out]
        n207 = Build Array (concatenate)("Select the test to run...", w319) -> (w318:string[])
        n208 = property on="Test Name" class="Ring (strict)"("Strings []"=w318) -> ()  [unwired: 2 in, 2 out]
      }
      event "Test Name": Value Change {
        w321 = FALSE ("Visible")
        # "Tell the robot the test name to run"
        n209 = event-data() -> ("NewVal"=w325:u16)  [unwired: 1 in]
        n210 = property on="Test Name" class="Ring (strict)"() -> ("Strings []"=w326:string[])  [unwired: 2 in, 2 out]
        n211 = local write "Progress"(T5 {"Test Progress"=0, "Test Progress Text"=""} ("Progress")) -> ()
        n212 = Index Array(array=w326, index=w325) -> (element=w324:string)
        n213 = call <vilib>:"NT Write String.vi"("String"=w324, "Name"="TestMode/TestName") -> ()  [unwired: 9 in, 1 out]
        n214 = property on="Progress" class="Clust (strict)"("Visible"=TRUE) -> ()  [unwired: 2 in, 2 out]
        n215 = property on="Motor" class="Clust (strict)"("Visible"=w321) -> ()  [unwired: 2 in, 2 out]
        n216 = property on="Test Slider" class="Slide (strict)"("Visible"=w321) -> ()  [unwired: 2 in, 2 out]
        n217 = property on="On/Off" class="Bool (strict)"("Visible"=w321) -> ()  [unwired: 2 in, 2 out]
        n218 = property on="Rev/Fwd" class="Clust (strict)"("Visible"=w321) -> ()  [unwired: 2 in, 2 out]
        n219 = property on="Test Ring" class="Ring (strict)"("Visible"=w321) -> ()  [unwired: 2 in, 2 out]
      }
      event "Select Auto": Mouse Enter {
        # "Populate the combo box with the list of autonomous options"
        n220 = event-data() -> ()  [unwired: 1 in, 1 out]
        n221 = call <vilib>:"NT Read String Array.vi"("Name"="Auto List") -> ("String Array"=w328:string[])  [unwired: 9 in, 1 out]
        n222 = property on="Select Auto" class="CmbBox"("Strings[]"=w328) -> ()  [unwired: 2 in, 2 out]
      }
      event "Select Auto": Value Change {
        # "User modified the Auto Selection. Write to NT variable so robot knows."
        n223 = event-data() -> ("NewVal"=w331:string)  [unwired: 1 in]
        n224 = call <vilib>:"NT Write String.vi"("String"=w331, "Name"="Auto Selector") -> ()  [unwired: 9 in, 1 out]
      }
      event "Command Selection": Value Change {
        # "Get the params and show in table"
        n225 = event-data() -> ("NewVal"=w337:i32)  [unwired: 1 in]
        n226 = property on="Command Selection" class="MCListbox (strict)"() -> ("ItemNames"=w335:string[][])  [unwired: 2 in, 2 out]
        n227 = call <vilib>:"WPI_DashboardUpdate Command Params.vi"("NewVal"=w337, "Commands"=w335, "Param Tbl"=w336) -> ()  [unwired: 8 in, 1 out]
      }
      event "Execute Command": Value Change {
        # "Started one, Unique ID holds\nresponse"
        n228 = event-data() -> ()  [unwired: 1 in, 1 out]
        n229 = property on="Command Selection" class="MCListbox (strict)"() -> ("ItemNames"=w348:string[][])  [unwired: 2 in, 2 out]
        n230 = Index Array(array=w348, index (row)="Command Selection", index (col)=0) -> (element=w346:string)
        n231 = call <vilib>:"Invoke Commands.vi"("Command Params"="Command Params", "Function Name"=w346) -> ("Params"=w342:u8, "Started"=w341:bool)  [unwired: 7 in, 1 out]
        n232 = Array Subset(array="Command Params", length (row)=w342) -> (w343:string[][])  [unwired: 3 in]
        n233 = Select(t="Executing" ("Cmd Status"), s=w341, f="" ("Cmd Status")) -> (s? t:f=→"Cmd Status":string)
      }
      event "Command Selection": Double Click {
        n234 = event-data() -> ("Row"=w356:i32)  [unwired: 1 in]
        n235 = property on="Command Selection" class="MCListbox (strict)"() -> ("ItemNames"=w359:string[][])  [unwired: 2 in, 2 out]
        n236 = local read "Command Params"() -> (w355:string[][])
        n237 = Index Array(array=w359, index (row)=w356, index (col)=0) -> (element=w357:string)
        n238 = call <vilib>:"Invoke Commands.vi"("Command Params"=w355, "Function Name"=w357) -> ("Params"=w354:u8, "Started"=w349:bool)  [unwired: 7 in, 1 out]
        n239 = Array Subset(array=w355, length (row)=w354) -> (w353:string[][])  [unwired: 3 in]
        n240 = Select(t="Executing" ("Cmd Status"), s=w349, f="" ("Cmd Status")) -> (s? t:f=w350:string)
        n241 = local write "Cmd Status"(w350) -> ()
      }
      event "CheckList": Double Click {
        # "Shift clears all"
        # "Update symbols on the listbox"
        n242 = event-data() -> ("PlatMods.Shift"=w361:bool, "Row"=w363:i32)  [unwired: 1 in]
        n243 = case shown="True" w361 {
          tunnel: w363 -> [w367 _]
          tunnel: 1 -> [w366 _]
          frame False {
            n244 = property on="CheckList" class="LstBox (strict)"() -> ("Item Symbols"=w365:i32[])  [unwired: 2 in, 2 out]
            n245 = Replace Array Subset(array=w365, new element=w366, index=w367) -> (w364:i32[])
            n246 = property on="CheckList" class="LstBox (strict)"("Item Symbols"=w364) -> ()  [unwired: 2 in, 2 out]
          }
          frame True {
            w368 = 0 ("Top Row")
            n247 = property on="CheckList" class="LstBox (strict)"() -> ("Number of Rows"=w370:u32)  [unwired: 2 in, 2 out]
            n248 = Initialize Array(0, w370) -> (w369:i32[])
            n249 = property on="CheckList" class="LstBox (strict)"("Top Row"=w368, "Value"=w368, "Item Symbols"=w369) -> ()  [unwired: 2 in, 2 out]
          }
        }
      }
      event "CheckList": Key Down {
        # "Update symbols on the listbox\nLeft and right keys check and uncheck"
        n250 = event-data() -> ("VKey"=w374:T17)  [unwired: 1 in]
        n251 = case shown="\"Left\", \"Right\"" w374 {
          selector: w374 -> [w379 _]
          tunnel: eventvkey."Left" ("VKey") -> [w377 _]
          frame "Left", "Right" {
            n252 = Equal?(x=w377, y=w379) -> (x = y?=w378:bool)
            n253 = Select(t=0, s=w378, f=1) -> (s? t:f=w380:i32)
            n254 = property on="CheckList" class="LstBox (strict)"() -> ("Item Symbols"=w383:i32[])  [unwired: 2 in, 2 out]
            n255 = Replace Array Subset(array=w383, new element=w380, index="CheckList") -> (w382:i32[])
            n256 = property on="CheckList" class="LstBox (strict)"("Item Symbols"=w382) -> ()  [unwired: 2 in, 2 out]
          }
          frame Default {
          }
        }
      }
      event "Motor.Enable": Value Change {
        # "When the test mode otor enable helper is set, update that\ntree row item's value"
        n257 = event-data() -> ("NewVal"=w389:bool)  [unwired: 1 in]
        n258 = Unbundle("Motor") -> ("Value"=w388:dbl)  [unwired: 1 out]
        n259 = Select(t=w388, s=w389, f=0.0) -> (s? t:f=w386:dbl)
        n260 = call <vilib>:"NT Write Number.vi"("Numeric"=w386, "Name"=w385) -> ()  [unwired: 9 in, 1 out]
      }
      event "Test Slider": Value Change {
        # "When the test mode slider helper is set, update that\ntree row item's value"
        n261 = event-data() -> ("NewVal"=w392:dbl)  [unwired: 1 in]
        n262 = call <vilib>:"NT Write Number.vi"("Numeric"=w392, "Name"=w393) -> ()  [unwired: 9 in, 1 out]
      }
      event "On/Off": Value Change {
        # "When the test mode on/off helper value is set, update that\ntree row item's value"
        n263 = event-data() -> ("NewVal"=w397:bool)  [unwired: 1 in]
        n264 = Boolean To (0,1)(Boolean=w397) -> (0, 1=w396:i16)
        n265 = call <vilib>:"NT Write Number.vi"("Numeric"=w396, "Name"=w395) -> ()  [unwired: 9 in, 1 out]
      }
      event "Rev/Fwd": Value Change {
        # "When the test mode helper value for relays is set, update that\ntree row item's value"
        n266 = event-data() -> ("NewVal.Forward"=w405:bool, "NewVal.Reverse"=w404:bool)  [unwired: 1 in]
        n267 = Boolean To (0,1)(Boolean=w405) -> (0, 1=w401:i16)
        n268 = Boolean To (0,1)(Boolean=w404) -> (0, 1=w403:i16)
        n269 = Negate(x=w403) -> (-x=w402:i16)
        n270 = Add(x=w401, y=w402) -> (x+y=w400:i16)
        n271 = call <vilib>:"NT Write Number.vi"("Numeric"=w400, "Name"=w399) -> ()  [unwired: 9 in, 1 out]
      }
      event "Test Ring": Value Change {
        # "When a test mode helper value is selected from the ring,\nset the tree item's variable to the string value"
        n272 = event-data() -> ("NewVal"=w409:u16)  [unwired: 1 in]
        n273 = property on="Test Ring" class="Ring (strict)"() -> ("Strings []"=w410:string[])  [unwired: 2 in, 2 out]
        n274 = Index Array(array=w410, index=w409) -> (element=w408:string)
        n275 = call <vilib>:"NT Write String.vi"("String"=w408, "Name"=w407) -> ()  [unwired: 9 in, 1 out]
      }
      event "Rec Mode": Value Change {
        # "Update globals for recording mode and path to read log from.\nClear when logging and let NetworkTables set path for vision to\nuse."
        n276 = event-data() -> ("NewVal"=w421:enum32{"Stop", "Record", "Playback"})  [unwired: 1 in]
        n277 = global write "WPI_DashboardLogging Global.vi" "Logging Filename"(path "") -> ()
        n278 = global write "WPI_DashboardLogging Global.vi" "Recording"(w421) -> ()
        n279 = case shown="\"Playback\"" w421 {
          tunnel: w420 -> [_ w423 w432]
          tunnel: [_ _ w431] -> w418
          tunnel: [_ _ w430] -> _
          tunnel: w416 -> [_ _ w428]
          tunnel: cluster{i32, i32} {-250, 170} -> [_ _ w427]
          tunnel: [_ _ T18 {"Image Size"=TRUE, "Image Type"=TRUE, "Pixel Value"=TRUE, "ROI Information"=TRUE, "Zoom Factor"=FALSE} ("Image Information Shown:All Elements")] -> w411
          tunnel: [_ _ TRUE ("Zoom Factor")] -> w412
          tunnel: w414 -> [_ _ w424]
          frame Default {
          }
          frame "Stop", "Record" {
            # "Place Window too"
            n280 = invoke class="VI" method="FP.Close"(reference=w423) -> (reference out=w422:refnum<vi>)  [unwired: 2 in, 2 out]
            n281 = invoke class="VI" method="Abort VI"(reference=w422) -> ()  [unwired: 2 in, 3 out]
          }
          frame "Playback" {
            n282 = call "Open Playback Panel.vi"("Offset"=w427, "DB VI Ref"=w428, "Playback in"=w432) -> ("Playback out"=w429:refnum<vi>)  [unwired: 8 in]
            n283 = register-events(w429, w424) -> (reference out=w431:refnum<event-registration>, error out=w430:errorcluster)  [unwired: 2 in]
          }
        }
        n284 = property on="Camera Image Right" class="ImageControl"("Image Information Shown"=w411, "Image Information Visible"=w412) -> ()  [unwired: 2 in, 2 out]
        n285 = property on="Camera Image" class="ImageControl"("Image Information Shown"=w411, "Image Information Visible"=w412) -> ()  [unwired: 2 in, 2 out]
        n286 = call <vilib>:"WPI_DashboardNT Log FieldName Cache.vi"("Operation"=enum16{"Lookup/Add", "Index", "Clear"}."Clear") -> ()  [unwired: 8 in, 3 out]
      }
      event Panel Close {
        w434 = enum32{"Stop", "Record", "Playback"}."Stop" ("Rec Mode")
        # "Playback window has been closed, abort"
        n287 = event-data() -> ()  [unwired: 1 in, 4 out]
        n288 = local write "Rec Mode"(w434) -> ()
        n289 = global write "WPI_DashboardLogging Global.vi" "Recording"(w434) -> ()
      }
      event Panel Close {
        # "Abort playback window and ourself"
        n290 = event-data() -> ()  [unwired: 1 in, 4 out]
        n291 = invoke class="VI" method="FP.Close"(reference=w438) -> (reference out=w437:refnum<vi>)  [unwired: 2 in, 2 out]
        n292 = invoke class="VI" method="Abort VI"(reference=w437) -> (error out=w436:errorcluster)  [unwired: 2 in, 2 out]
        n293 = invoke class="VI" method="Abort VI"(error in=w436) -> ()  [unwired: 2 in, 3 out]
      }
      event User Event {
        n294 = event-data() -> ("IDs"=w445:cluster{"RPC field ID":u16, "Unique ID":u16}, "String"=w444:string)  [unwired: 1 in]
        n295 = Bundle("IDs"=w445, "String"=w444) -> (w443:T8)  [unwired: 1 in]
        n296 = call <vilib>:"Retrieve RPC Response.vi"("RPC Response"=w443) -> ("Output"=w441:string[][])  [unwired: 10 in]
        n297 = Build Array (concatenate)(w439, w441) -> (w440:string[][])
        n298 = local write "Command Params"(w440) -> ()
        n299 = local write "Cmd Status"("" ("Cmd Status")) -> ()
      }
      event "Tree": Double Click {
        n300 = event-data() -> ("PlatMods"=w451:T21, "Tag"=w448:string)  [unwired: 1 in]
        n301 = Unbundle(w451) -> ("Shift"=w450:bool)  [unwired: 4 out]
        n302 = String Subset(string=w448, length (rest)=1 ("length (rest)")) -> (substring=w447:string)  [unwired: 1 in]
        n303 = Not(x=w450) -> (.not. x?=w449:bool)
        n304 = case shown="\"/\"" w447 {
          tunnel: w448 -> [_ w454]
          tunnel: w449 -> [_ w453]
          frame Default {
          }
          frame "/" {
            n305 = call <vilib>:"NT Update Persistence.vi"("Persistence"=w453, "Name"=w454) -> ()  [unwired: 9 in, 1 out]
          }
        }
      }
    }
  }
  n306 = while {
    tunnel: w61 -> [w456]
    i -> [w459]
    stop <- FALSE stop-if-true
    n307 = Wait (ms)(milliseconds to wait=u32 100) -> ()  [unwired: 1 out]
    n308 = case shown="\"Playback\"" "Rec Mode" {
      tunnel: w459 -> [_ _ w474]
      tunnel: [u32 2829099 ("Base Color") u32 11141120 ("Target Color") w463] -> w455
      frame "Stop", Default {
        # "Reset the color, extra updates don't cost much"
      }
      frame "Record" {
      }
      frame "Playback" {
        # "Playback"
        n309 = Quotient & Remainder(x=w474, y=u32 50 ("milliseconds to wait")) -> (x-y*floor(x/y)=w470:u32)  [unwired: 1 out]
        n310 = Divide(x=w470, y=u32 50 ("milliseconds to wait")) -> (x/y=w467:dbl)
        n311 = Multiply(x=6.283185307179586, y=w467) -> (x*y=w472:dbl)
        n312 = Sine(x=w472) -> (sin(x)=w471:dbl)
        n313 = Absolute Value(x=w471) -> (abs(x)=w464:dbl)
        n314 = call "Interpolate RGB Color.vi"("Proportion"=w464, "Target Color"=u32 30976, "Base Color"=u32 2829099) -> ("Result Color"=w463:u32)  [unwired: 8 in]
      }
    }
    n315 = property class="Pane"(reference=w456, "PaneColor"=w455) -> ()  [unwired: 1 in, 2 out]
  }
  n316 = local write "Dashboard Tab"(T1."Drive" ("Dashboard Tab")) -> ()
  n317 = property on="On/Off" class="Bool (strict)"("Visible"=w34) -> ()  [unwired: 2 in, 2 out]
  n318 = property on="Motor" class="Clust (strict)"("Visible"=w34) -> ()  [unwired: 2 in, 2 out]
  n319 = property on="Progress" class="Clust (strict)"("Visible"=w34) -> ()  [unwired: 2 in, 2 out]
  n320 = property on="Test Ring" class="Ring (strict)"("Visible"=w34) -> ()  [unwired: 2 in, 2 out]
  n321 = property on="Rev/Fwd" class="Clust (strict)"("Visible"=w34) -> ()  [unwired: 2 in, 2 out]
  n322 = while {
    tunnel: u16 1741 ("timeout ms (25000)") -> [w476]
    stop <- FALSE stop-if-true
    n323 = TCP Create Listener(10:w476) -> (0:w475:errorcluster, 3:w477:refnum<k5>)  [unwired: 4 in, 1 out]
    n324 = case shown="No Error" w475 {
      selector: w475 -> [w479 _]
      tunnel: w477 -> [w480 _]
      frame No Error {
        n325 = while {
          tunnel: w480 -> [w483]
          tunnel: w479 -> [w482]
          stop <- FALSE stop-if-true
          n326 = TCP Wait On Listener(8:w482, 11:w483) -> (0:w484:errorcluster, 4:w485:refnum<k5>)  [unwired: 2 in, 3 out]
          n327 = local write "TCP"(w485) -> ()
          n328 = case shown="No Error" w484 {
            frame No Error {
            }
            frame Error {
              n329 = Wait (ms)(milliseconds to wait=u32 1000) -> ()  [unwired: 1 out]
            }
          }
        }
      }
      frame Error {
        n330 = Wait (ms)(milliseconds to wait=u32 1000) -> ()  [unwired: 1 out]
      }
    }
  }
  n331 = local write "Command Selection"(u16 0 ("milliseconds to wait")) -> ()
  n332 = local write "Command Params"(string[][] [] ("Command Params")) -> ()
  n333 = global write "WPI_DashboardLogging Global.vi" "Recording"(w55) -> ()
  n334 = local write "Rec Mode"(w55) -> ()
  n335 = disable-structure shown="Disabled" {
    frame Disabled {
      n336 = while {
        stop <- FALSE stop-if-true
        n337 = call <vilib>:"Application Directory.vi"() -> ("Application Directory"=w496:path)
        n338 = Wait (ms)(milliseconds to wait=u32 1000) -> ()  [unwired: 1 out]
        n339 = Strip Path(path=w496) -> (stripped path=w489:path)  [unwired: 1 out]
        n340 = local read "Select Auto"() -> (w492:string)
        n341 = Strip Path(path=w489) -> (stripped path=w490:path)  [unwired: 1 out]
        n342 = Equal?(x=w492, y="Select Autonomous ...") -> (x = y?=w491:bool)
        n343 = Build Path(base path=w490, name or relative path="PathPictures") -> (appended path=w493:path)
        n344 = case shown="False" w491 {
          tunnel: w493 -> [w503 w507]
          tunnel: [w501 w506] -> w488
          tunnel: w492 -> [w502 _]
          frame False {
            n345 = Concatenate Strings(w502, ".jpg" ("string")) -> (w505:string)
            n346 = Build Path(base path=w503, name or relative path=w505) -> (appended path=w501:path)
          }
          frame True {
            n347 = Build Path(base path=w507, name or relative path="2019Field.jpg") -> (appended path=w506:path)
          }
        }
        n348 = call <vilib>:"Read JPEG File.vi"("path to JPEG file"=w488) -> ("image data"=w497:T22)  [unwired: 8 in, 2 out]
        n349 = call <vilib>:"Draw Flattened Pixmap.vi"("image data"=w497) -> ("new picture"=w498:picture)  [unwired: 8 in]
      }
    }
    frame Enabled {
    }
  }
  n350 = call "Secondary Moniter.vi"() -> ()  [unwired: 1 in]
  n351 = while {
    stop <- FALSE stop-if-true
    n352 = Wait (ms)(milliseconds to wait=u32 100) -> ()  [unwired: 1 out]
    n353 = call-poly <vilib>:"NT Read Value.vi"("Name"="Elevator_Position") -> ("Numeric"=w543:dbl)  [unwired: 9 in, 1 out]
    n354 = call-poly <vilib>:"NT Read Value.vi"("Name"="Elevator_Desired") -> ("Numeric"=w544:dbl)  [unwired: 9 in, 1 out]
    n355 = Bundle("Numeric"=w543, "Numeric"=w544) -> (→"Elevator\nPosition":cluster{"Numeric":dbl, "Numeric":dbl})  [unwired: 1 in]
    n356 = call-poly <vilib>:"NT Read Value.vi"("Name"="Manipulator2") -> ("Boolean Array"=w536:bool[])  [unwired: 9 in, 1 out]
    n357 = call-poly <vilib>:"NT Read Value.vi"("Name"="Manipulator1") -> ("Boolean Array"=w537:bool[])  [unwired: 9 in, 1 out]
    n358 = Index Array(array=w537) -> (element #1=→"Boolean 9":bool, element #2=→"Boolean 2":bool, element #3=→"Boolean 8":bool, element #4=→"Boolean 17":bool, element #5=→"Boolean 6":bool, element #6=→"Boolean":bool, element #7=→"Boolean 4":bool, element #8=→"Boolean":bool, element #9=→"Boolean":bool, element #10=→"Boolean 5":bool, element #11=→"Boolean 3":bool, element #12=→"Boolean":bool)  [unwired: 12 in]
    n359 = Index Array(array=w536) -> (element #1=→"Boolean 12":bool, element #2=→"Boolean 15":bool, element #3=→"Boolean 11":bool, element #4=→"Boolean 13":bool, element #5=→"Boolean 10":bool, element #6=→"Boolean 16":bool, element #7=→"Boolean 14":bool)  [unwired: 7 in]
    n360 = call-poly <vilib>:"NT Read Value.vi"("Name"="Hatch_Open") -> ("Boolean"=→"Hatch Open":bool)  [unwired: 9 in, 1 out]
    n361 = call-poly <vilib>:"NT Read Value.vi"("Name"="Hatch_Close") -> ("Boolean"=→"Hatch Close":bool)  [unwired: 9 in, 1 out]
    n362 = call-poly <vilib>:"NT Read Value.vi"("Name"="Ball_In") -> ("Boolean"=→"Ball In":bool)  [unwired: 9 in, 1 out]
    n363 = call-poly <vilib>:"NT Read Value.vi"("Name"="Ball_Out") -> ("Boolean"=→"Ball Out":bool)  [unwired: 9 in, 1 out]
  }
